vi "Process_Exposures_Table.vi"(2 "shot names":string[](array[string]), 3 "sequence names":string[](array[string])) -> (0 "list":string[][](array[string]), 1 "sequences":T1(array[cluster]))   [LabVIEW 2012]
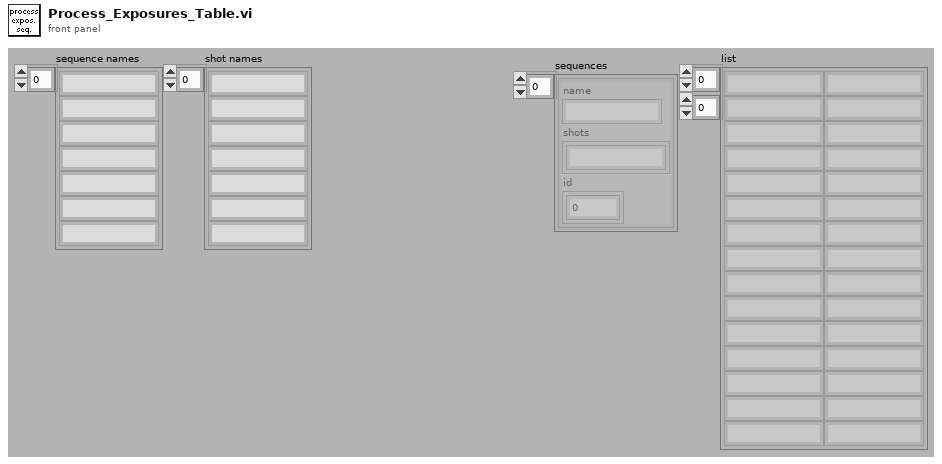
[diagram p1: front panel]
types:
  T1 = cluster{"name":string, "shots":string[], "id":i32[]}[]
  T2 = cluster{"name":string, "shots":string[], "id":i32[]}
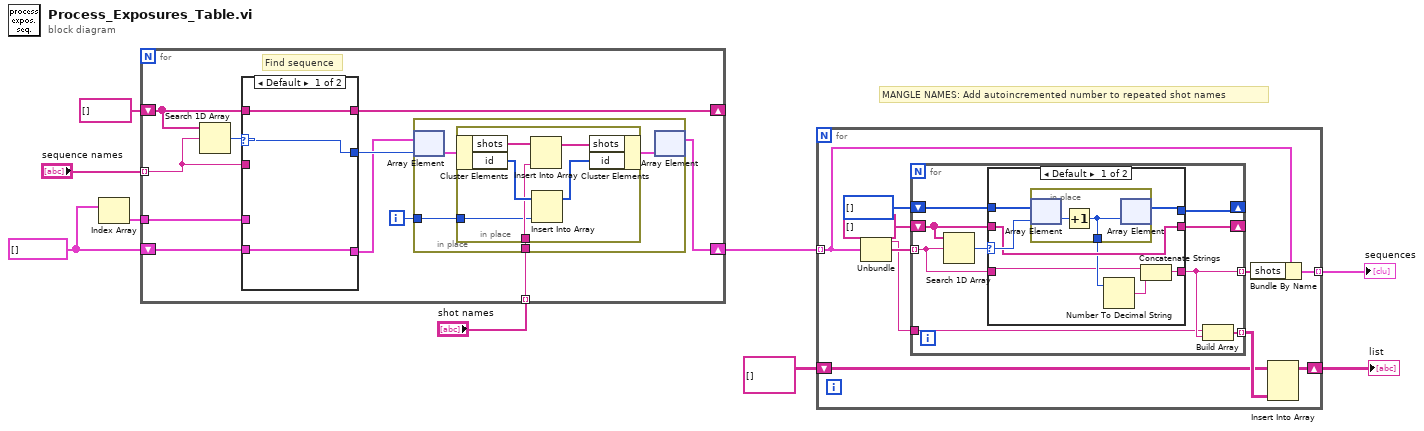
[diagram p0: block diagram]
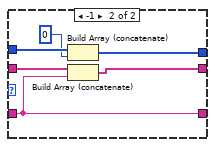
[diagram p2: hidden frame]
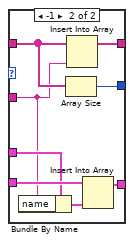
[diagram p3: hidden frame]
diagram:
  w5 = T1 []
  # "MANGLE NAMES: Add autoincremented number to repeated shot names"
  n1 = Index Array(array=w5) -> (element=w6:T2)  [unwired: 1 in]
  n2 = for {
    shift-right: [w18] -> _
    shift-left: string[] [] -> [w19]
    shift-right: [w16] -> w4
    shift-left: w5 -> [w14]
    tunnel: w6 -> [w12]
    tunnel: "sequence names" -> [w11] mode=indexing
    tunnel: "shot names" -> [w10] mode=indexing
    i -> [w15]
    # "Find sequence"
    n3 = Search 1D Array(1D array=w19, element=w11) -> (index of element=w20:i32)  [unwired: 1 in]
    n4 = case shown="Default" w20 {
      selector: w20 -> [w32 _]
      tunnel: w11 -> [_ w34]
      tunnel: w19 -> [w33 w40]
      tunnel: [w33 w41] -> w18
      tunnel: [w32 w39] -> w17
      tunnel: w14 -> [w31 w38]
      tunnel: [w31 w37] -> w13
      tunnel: w12 -> [_ w36]
      frame Default {
      }
      frame -1 {
        n5 = Bundle By Name(cluster=w36, "name"=w34) -> (w35:T2)
        n6 = Array Size(array=w40) -> (size(s)=w39:i32)
        n7 = Insert Into Array(array=w40, new element=w34) -> (w41:string[])  [unwired: 1 in]
        n8 = Insert Into Array(array=w38, new element=w35) -> (w37:T1)  [unwired: 1 in]
      }
    }
    n9 = in-place {
      in-place-border: w10 -> [w22]
      in-place-border: w15 -> [w21]
      n10 = in-place-array #1(w13, w17) -> (w24:T2)
      n11 = in-place {
        in-place-border: w22 -> [w26]
        in-place-border: w21 -> [w25]
        n12 = in-place-cluster #2(w24) -> ("shots"=w30:string[], "id"=w28:i32[])
        n13 = Insert Into Array(array=w30, new element=w26) -> (w29:string[])  [unwired: 1 in]
        n14 = Insert Into Array(array=w28, new element=w25) -> (w27:i32[])  [unwired: 1 in]
        n15 = in-place-cluster #2("shots"=w29, "id"=w27) -> (w23:T2)
      }
      n16 = in-place-array #1(w23) -> (w16:T1)  [unwired: 1 out]
    }
  }
  n17 = for {
    tunnel: w4 -> [w48] mode=indexing
    tunnel: [w47] -> w3 mode=indexing
    shift-right: [w42] -> w1
    shift-left: string[][] [] -> [w43]
    n18 = Unbundle(w48) -> ("name"=w45:string, "shots"=w51:string[])  [unwired: 1 out]
    n19 = for {
      tunnel: w51 -> [w59] mode=indexing
      tunnel: [w54] -> w46 mode=indexing
      shift-right: [w56] -> _
      shift-left: i32[] [] -> [w57]
      shift-right: [w55] -> _
      shift-left: string[] [] -> [w58]
      tunnel: w45 -> [w53]
      tunnel: [w52] -> w44 mode=indexing
      n20 = Search 1D Array(1D array=w58, element=w59) -> (index of element=w60:i32)  [unwired: 1 in]
      n21 = case shown="Default" w60 {
        selector: w60 -> [w67 _]
        tunnel: w59 -> [w63 w71]
        tunnel: w58 -> [w66 w76]
        tunnel: w57 -> [w68 w75]
        tunnel: [w65 w73] -> w56
        tunnel: [w66 w72] -> w55
        tunnel: [w62 w71] -> w54
        frame Default {
          n22 = in-place {
            in-place-border: [w69] -> w64
            n23 = in-place-array #3(w68, w67) -> (w70:i32)
            n24 = Increment(x=w70) -> (x+1=w69:i32)
            n25 = in-place-array #3(w69) -> (w65:i32[])  [unwired: 1 out]
          }
          n26 = Number To Decimal String(number=w64) -> (decimal integer string=w61:string)  [unwired: 1 in]
          n27 = Concatenate Strings(w63, w61) -> (w62:string)
        }
        frame -1 {
          n28 = Build Array (concatenate)(w75, 0) -> (w73:i32[])
          n29 = Build Array (concatenate)(w76, w71) -> (w72:string[])
        }
      }
      n30 = Build Array(w53, w54) -> (w52:string[])
    }
    n31 = Bundle By Name(cluster=w48, "shots"=w46) -> (w47:T2)
    n32 = Insert Into Array(array=w43, new element=w44) -> (w42:string[][])  [unwired: 2 in]
  }
  "sequences" <- w3
  "list" <- w1
